vi "sub_test-finish.vi"   [LabVIEW 2019]
uses:
  SubVIs/common/_ctrl/system-status.ctl
types:
  T1 = typedef "system-status.ctl" = enum16{"Initial", "Update", "Clear", "Read"}
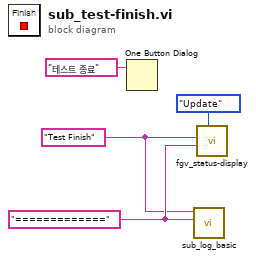
[diagram p0: block diagram]
diagram:
  w4 = "=============" ("desc")
  w3 = "Test Finish" ("Title")
  n1 = One Button Dialog(message="테스트 종료") -> ()  [unwired: 1 in, 1 out]
  n2 = call "sub_log_basic.vi"("desc"=w4, "Title"=w3) -> ()  [unwired: 9 in, 1 out]
  n3 = call "fgv_status-display.vi"("Mode"=system-status."Update", "detail"=w4, "title"=w3) -> ()  [unwired: 8 in, 1 out]
